vi "Index.vi"() -> ()   [LabVIEW 2016]
panel:
  out "Index":dbl
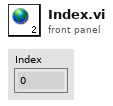
[diagram p1: front panel]
diagram:
